vi "Configure Declination Angle Input For True North.vi"(8 "error in (no error)":errorcluster, 10 "Declination Angle ( 0 degrees)":i32, 11 "VISA resource name":refnum<visa-resource-name>) -> (0 "error out":errorcluster, 3 "VISA resource out":refnum<visa-resource-name>)   [LabVIEW 2011, in "Ocean Server OS4000.lvlib"]
doc: "Set a fixed heading offset to be applied to all heading output data. In most cases this is used to adjust for local compass deviation in your area.\n\nThis information can be found on the web using the World Magnetic Model and you local LATITUDE,LONGITUDE. Enter Declination angle to create offset for compass\nAzimuth. Value is 10x degrees. Example: -103=-10.3 degrees, 152=15.2 degrees.\n\nhttp://en.wikipedia.org/wiki/Magnetic_declination"
uses:
  Ocean Server OS4000.lvlib
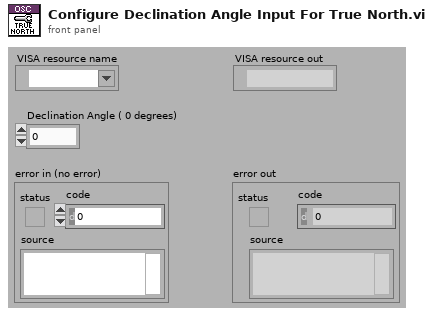
[diagram p1: front panel]
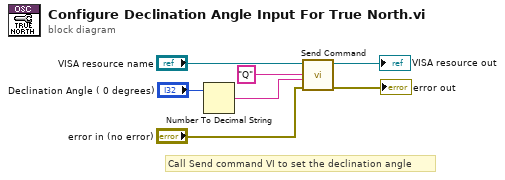
[diagram p0: block diagram]
diagram:
  # "Call Send command VI to set the declination angle"
  n1 = Number To Decimal String(number="Declination Angle ( 0 degrees)") -> (decimal integer string=w4:string)  [unwired: 1 in]
  n2 = call "Send Command.vi"("error in (no error)"="error in (no error)", "Value"=w4, "Message"="Q", "VISA resource name"="VISA resource name") -> ("error out"=→"error out":errorcluster, "VISA resource out"=→"VISA resource out":refnum<visa-resource-name>)  [unwired: 6 in]
